vi "CalculateFlux.vi"(9 "Ion Charge State":u8, 10 "Irradiation Area (cm^2)":dbl, 11 "Beam Current (A)":dbl) -> (3 "Flux (ions/s * cm^2)":dbl)   [LabVIEW 2012]
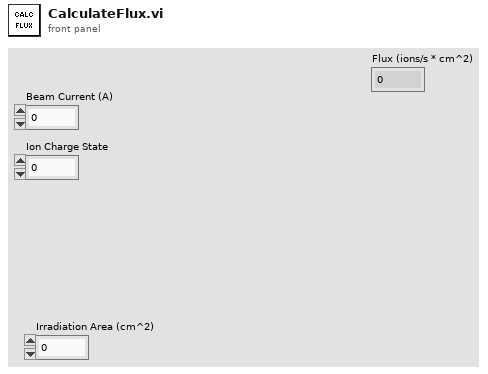
[diagram p1: front panel]
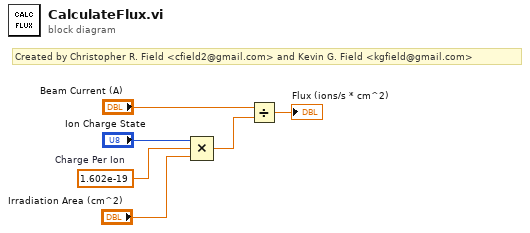
[diagram p0: block diagram]
diagram:
  w5 = 1.602e-19  # Charge Per Ion
  # "Created by Christopher R. Field <cfield2@gmail.com> and Kevin G. Field <kgfield@gmail.com>"
  n1 = Compound Arithmetic op=MULTIPLY("Ion Charge State", w5, "Irradiation Area (cm^2)") -> (w2:dbl)
  n2 = Divide(x="Beam Current (A)", y=w2) -> (x/y=→"Flux (ions/s * cm^2)":dbl)
